vi "Send 10 -100.vi"() -> ()   [LabVIEW 2015]
panel:
  out "100 byte":i32[][](array[numeric])
  out "Time":u32
  in  "stop":bool
  out "Delay (ms)":u32
  out "Average Delay (ms)":dbl
  out "Tries":u32
  out "10 byte":u64[](array[numeric])
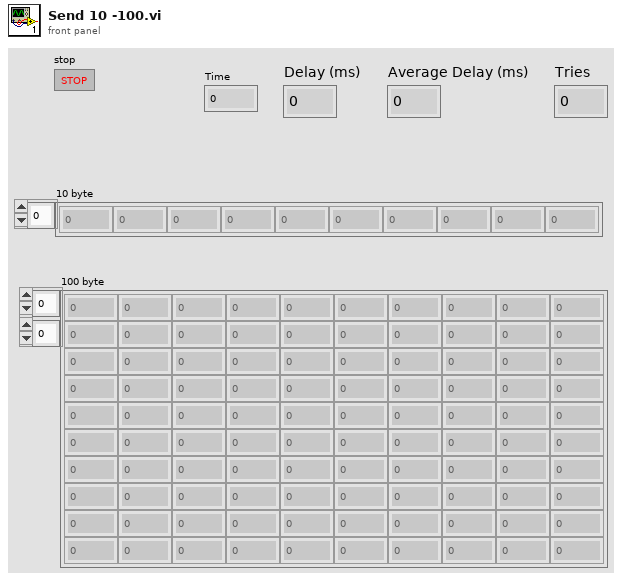
[diagram p1: front panel]
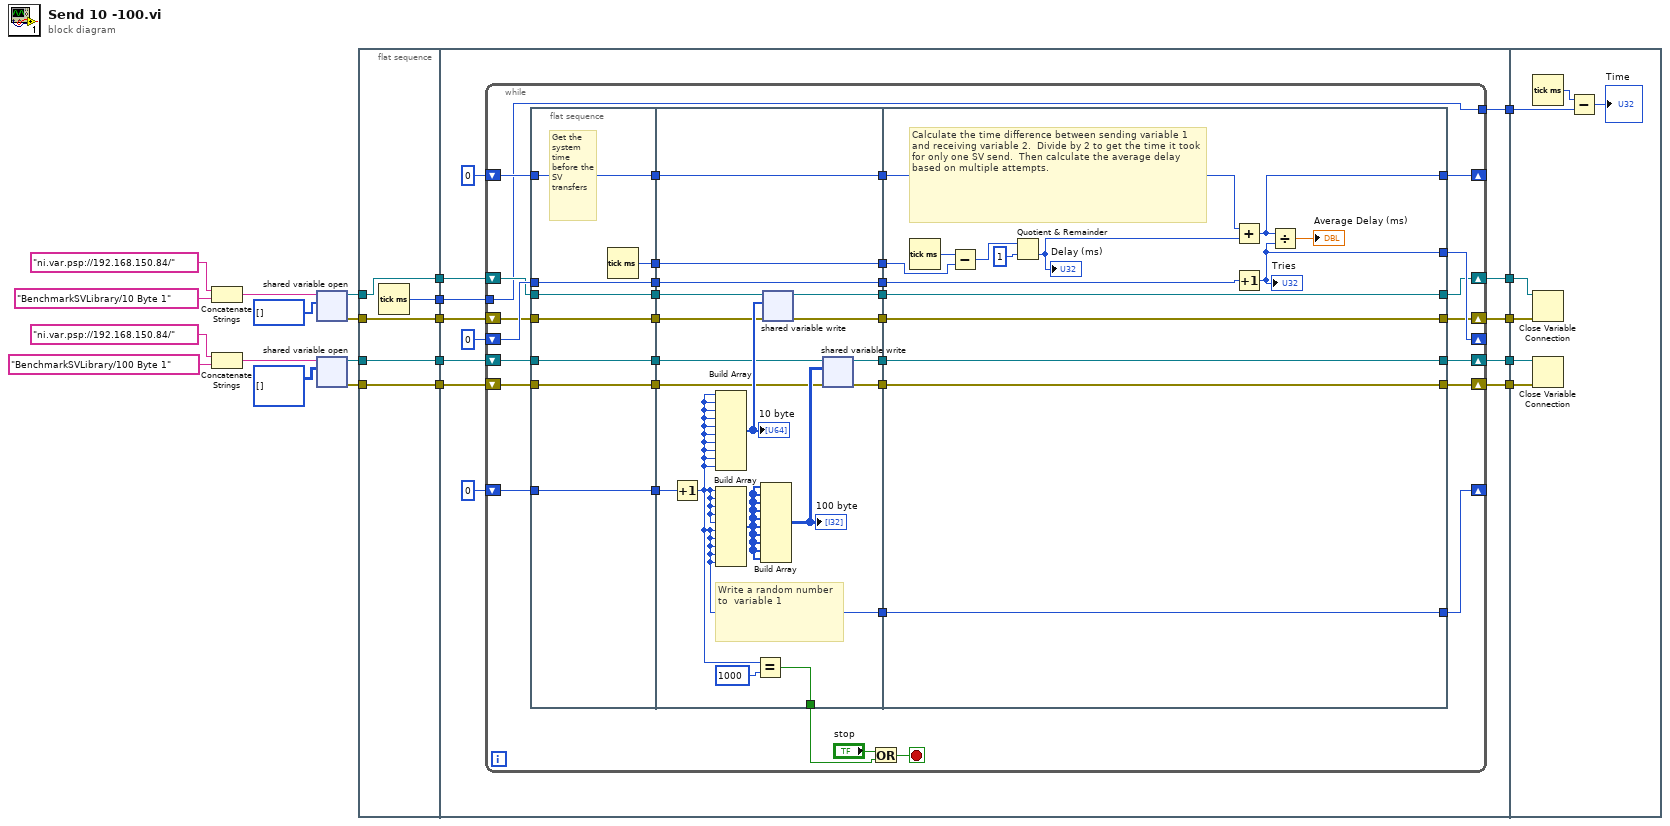
[diagram p0: block diagram]
diagram:
  n1 = Concatenate Strings("ni.var.psp://192.168.150.84/" ("string"), "BenchmarkSVLibrary/10 Byte 1") -> (w15:string)
  n2 = Concatenate Strings("ni.var.psp://192.168.150.84/" ("string"), "BenchmarkSVLibrary/100 Byte 1") -> (w10:string)
  n3 = shared-variable-open(w15, u64[] [] ("appended array")) -> (w13:refnum<k21>, w14:errorcluster)  [unwired: 2 in]
  n4 = shared-variable-open(w10, i32[][] [] ("appended array")) -> (w5:refnum<k21>, w3:errorcluster)  [unwired: 2 in]
  n5 = flat-sequence {
    tunnel: w13 -> [w26]
    tunnel: w14 -> [w27]
    tunnel: [w27] -> w22
    tunnel: [w26] -> w21
    tunnel: [w25] -> w20
    tunnel: [w24] -> w6
    tunnel: w5 -> [w24]
    tunnel: [w23] -> w4
    tunnel: w3 -> [w23]
    tunnel: [w35] -> w19
    tunnel: w22 -> [w37]
    tunnel: w21 -> [w36]
    tunnel: w20 -> [w34]
    tunnel: [w33] -> w18
    tunnel: [w32] -> w17
    tunnel: w6 -> [w31]
    tunnel: w4 -> [w30]
    tunnel: [w29] -> w2
    tunnel: [w28] -> w1
    tunnel: w19 -> [w120]
    tunnel: w18 -> [w119]
    tunnel: w17 -> [w118]
    tunnel: w2 -> [w117]
    tunnel: w1 -> [w116]
    frame #0 {
      n6 = Tick Count (ms)() -> (millisecond timer value=w25:u32)
    }
    frame #1 {
      n7 = while {
        shift-right: [w74] -> _
        shift-left: u32 0 -> [w68]
        shift-right: [w73] -> _
        shift-left: u32 0 -> [w69]
        shift-right: [w65] -> _
        shift-left: u64 0 -> [w66]
        shift-right: [w57] -> w33
        shift-left: w37 -> [w55]
        shift-right: [w52] -> w32
        shift-left: w36 -> [w50]
        tunnel: [w49] -> w35
        tunnel: w34 -> [w49]
        shift-right: [w44] -> w29
        shift-left: w31 -> [w47]
        shift-right: [w42] -> w28
        shift-left: w30 -> [w45]
        stop <- w64 stop-if-true
        n8 = flat-sequence {
          tunnel: [w80] -> w72
          tunnel: [w82] -> w71
          tunnel: [w81] -> w70
          tunnel: [w79] -> w67
          tunnel: [w78] -> w54
          tunnel: [w77] -> w53
          tunnel: w68 -> [w82]
          tunnel: w69 -> [w81]
          tunnel: w66 -> [w79]
          tunnel: w55 -> [w78]
          tunnel: w50 -> [w77]
          tunnel: [w76] -> w48
          tunnel: w47 -> [w76]
          tunnel: [w75] -> w46
          tunnel: w45 -> [w75]
          tunnel: [w100] -> w61
          tunnel: [w99] -> w60
          tunnel: [w98] -> w59
          tunnel: w72 -> [w100]
          tunnel: w71 -> [w99]
          tunnel: w70 -> [w98]
          tunnel: w67 -> [w97]
          tunnel: [w87] -> w58
          tunnel: [w95] -> w62
          tunnel: [w93] -> w56
          tunnel: w54 -> [w92]
          tunnel: w53 -> [w91]
          tunnel: [w90] -> w51
          tunnel: w48 -> [w86]
          tunnel: w46 -> [w85]
          tunnel: [w84] -> w43
          tunnel: [w83] -> w41
          tunnel: w61 -> [w114]
          tunnel: [w107] -> w74
          tunnel: w60 -> [w109]
          tunnel: [w106] -> w73
          tunnel: w59 -> [w113]
          tunnel: w58 -> [w105]
          tunnel: [w105] -> w65
          tunnel: [w104] -> w57
          tunnel: w56 -> [w104]
          tunnel: [w103] -> w52
          tunnel: w51 -> [w103]
          tunnel: [w102] -> w44
          tunnel: w43 -> [w102]
          tunnel: [w101] -> w42
          tunnel: w41 -> [w101]
          frame #0 {
            # "Get the system time before the SV transfers"
            n9 = Tick Count (ms)() -> (millisecond timer value=w80:u32)
          }
          frame #1 {
            # "Write a random number to  variable 1"
            n10 = Increment(x=w97) -> (x+1=w87:u64)
            n11 = Build Array(w87, w87, w87, w87, w87, w87, w87, w87, w87, w87) -> (w94:u64[])
            "10 byte" <- w94
            n12 = Build Array(w87, w87, w87, w87, w87, w87, w87, w87, w87, w87) -> (w89:u64[])
            n13 = Equal?(x=w87, y=u64 1000) -> (x = y?=w95:bool)
            n14 = Build Array(w89, w89, w89, w89, w89, w89, w89, w89, w89, w89) -> (w88:u64[][])
            "100 byte" <- w88
            n15 = shared-variable-write(w91, w92, w94) -> (w90:refnum<k21>, w93:errorcluster)
            n16 = shared-variable-write(w86, w85, w88) -> (w84:refnum<k21>, w83:errorcluster)
          }
          frame #2 {
            # "Calculate the time difference between sending variable 1 and receiving variable 2.  Divide by 2 to get the time it took for only one SV send.  Then calculate the average delay based on multiple attempts."
            n17 = Tick Count (ms)() -> (millisecond timer value=w115:u32)
            n18 = Subtract(x=w115, y=w114) -> (x-y=w112:u32)
            n19 = Quotient & Remainder(x=w112, y=u32 1) -> (floor(x/y)=w110:u32)  [unwired: 1 out]
            "Delay (ms)" <- w110
            n20 = Add(x=w109, y=w110) -> (x+y=w107:u32)
            n21 = Increment(x=w113) -> (x+1=w106:u32)
            "Tries" <- w106
            n22 = Divide(x=w107, y=w106) -> (x/y=→"Average Delay (ms)":dbl)
          }
        }
        n23 = Or(x="stop", y=w62) -> (x .or. y?=w64:bool)
      }
    }
    frame #2 {
      n24 = Tick Count (ms)() -> (millisecond timer value=w122:u32)
      n25 = Close Variable Connection(8:w119, 11:w118) -> ()  [unwired: 1 out]
      n26 = Close Variable Connection(8:w116, 11:w117) -> ()  [unwired: 1 out]
      n27 = Subtract(x=w122, y=w120) -> (x-y=→"Time":u32)
    }
  }
